vi "test_CCDSetAndGetFitParams.vi"(7 "Test should pass":bool=TRUE, 8 "error in":errorcluster, 9 "tear down connection":bool=TRUE, 10 "set-up a connection":bool=TRUE, 11 "device selection":enum16{"monochromator", "CCD", "SCD"}(ring)=enum."CCD") -> (0 "error out":errorcluster)   [LabVIEW 2023]
uses:
  Classes/CCD/CCD.lvclass
  C:/Projects/Horiba/horiba-labview-sdk/Source/Classes/GenericDevice/GenericDevice.lvclass
  <vilib>/addons/_JKI Toolkits/Caraya/classes/Assert/Assert Equal Value and Type_Variant.vi
  <vilib>/addons/_JKI Toolkits/Caraya/classes/Assert/Assert Not Error.vi
  <vilib>/addons/_JKI Toolkits/Caraya/classes/Assert/Assert Equal Value_Variant.vi
  <vilib>/addons/_JKI Toolkits/Caraya/classes/Test/Test.lvclass
  <vilib>/addons/_JKI Toolkits/Caraya/classes/Assert/Assert.lvclass
panel:
  out "fit parameters":string
  # "Connector Pane"
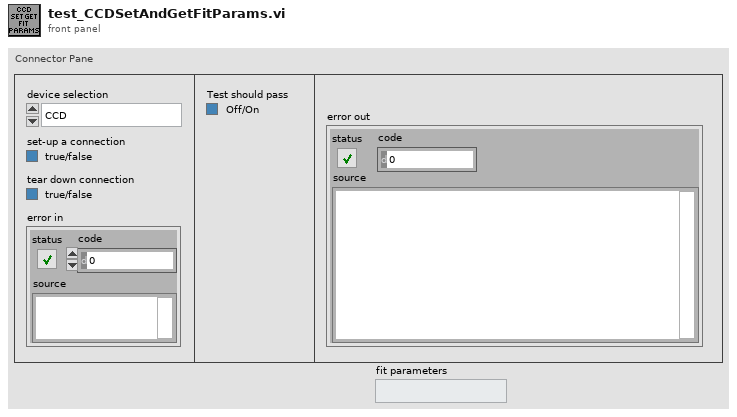
[diagram p1: front panel]
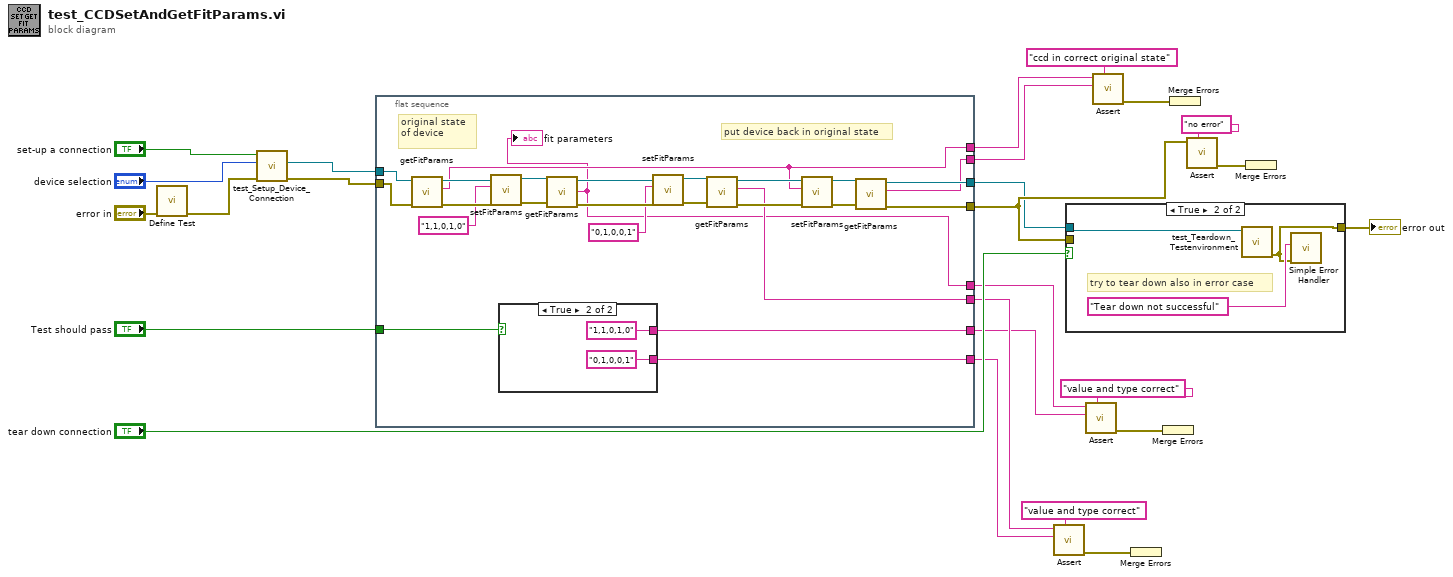
[diagram p0: block diagram]
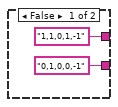
[diagram p2: hidden frame]
diagram:
  n1 = call <vilib>:"Define Test.vi"("error in (no error)"="error in") -> ("error out"=w3:errorcluster)  [unwired: 9 in, 1 out]
  n2 = call "test_Setup_Device_Connection.vi"("error in (no error)"=w3, "device selection"="device selection", "set-up a connection"="set-up a connection") -> ("error out"=w5:errorcluster, "CCD.lvclass"=w4:refnum<class "CCD.lvclass">)  [unwired: 5 in, 2 out]
  n3 = flat-sequence {
    tunnel: w5 -> [w46]
    tunnel: w4 -> [w47]
    tunnel: [w32] -> w16
    tunnel: "Test should pass" -> [w50]
    tunnel: [w39] -> w15
    tunnel: [w27] -> w14
    tunnel: [w49] -> w13
    tunnel: [w26] -> w12
    tunnel: [w48] -> w11
    tunnel: [w30] -> w8
    tunnel: [w31] -> w7
    frame #0 {
      # "put device back in original state"
      # "original state of device"
      n4 = call "getFitParams.vi"("error in (no error)"=w46, "CCD in"=w47) -> ("error out"=w38:errorcluster, "fit parameters"=w30:string, "CCD out"=w45:refnum<class "CCD.lvclass">)  [unwired: 7 in]
      n5 = call "setFitParams.vi"("error in (no error)"=w38, "fit parameters"="1,1,0,1,0", "CCD in"=w45) -> ("error out"=w37:errorcluster, "CCD out"=w44:refnum<class "CCD.lvclass">)  [unwired: 5 in, 2 out]
      n6 = case shown="True" w50 {
        tunnel: ["0,1,0,0,-1" "0,1,0,0,1"] -> w49
        tunnel: ["1,1,0,1,-1" "1,1,0,1,0"] -> w48
        frame False {
        }
        frame True {
        }
      }
      n7 = call "getFitParams.vi"("error in (no error)"=w37, "CCD in"=w44) -> ("error out"=w36:errorcluster, "fit parameters"=w26:string, "CCD out"=w43:refnum<class "CCD.lvclass">)  [unwired: 7 in]
      "fit parameters" <- w26
      n8 = call "setFitParams.vi"("error in (no error)"=w36, "fit parameters"="0,1,0,0,1", "CCD in"=w43) -> ("error out"=w35:errorcluster, "CCD out"=w42:refnum<class "CCD.lvclass">)  [unwired: 5 in, 2 out]
      n9 = call "getFitParams.vi"("error in (no error)"=w35, "CCD in"=w42) -> ("error out"=w34:errorcluster, "fit parameters"=w27:string, "CCD out"=w41:refnum<class "CCD.lvclass">)  [unwired: 7 in]
      n10 = call "setFitParams.vi"("error in (no error)"=w34, "fit parameters"=w30, "CCD in"=w41) -> ("error out"=w33:errorcluster, "CCD out"=w40:refnum<class "CCD.lvclass">)  [unwired: 5 in, 2 out]
      n11 = call "getFitParams.vi"("error in (no error)"=w33, "CCD in"=w40) -> ("error out"=w32:errorcluster, "fit parameters"=w31:string, "CCD out"=w39:refnum<class "CCD.lvclass">)  [unwired: 7 in]
    }
  }
  n12 = call-poly <vilib>:"Assert.vi"("Label"="value and type correct" ("Label (VI Title)"), "Y"=w13, "X"=w14) -> ("error out"=w24:errorcluster)  [unwired: 7 in, 1 out]
  n13 = case shown="True" "tear down connection" {
    tunnel: w15 -> [_ w57]
    tunnel: [w55 w56] -> w6
    tunnel: w16 -> [w55 _]
    frame False {
    }
    frame True {
      # "try to tear down also in error case"
      n14 = call "test_Teardown_Testenvironment.vi"("GenericDevice.lvclass"=w57) -> ("error out"=w56:errorcluster)  [unwired: 9 in, 1 out]
      n15 = call <vilib>:"Simple Error Handler.vi"("error source (\" \")"="Tear down not successful" ("error source (\" \")"), "error in (no error)"=w56) -> ()  [unwired: 3 in, 5 out]
    }
  }
  "error out" <- w6
  n16 = call-poly <vilib>:"Assert.vi"("Label"="value and type correct" ("Label (VI Title)"), "Y"=w11, "X"=w12) -> ("error out"=w23:errorcluster)  [unwired: 7 in, 1 out]
  n17 = call-poly <vilib>:"Assert.vi"("Label"="ccd in correct original state" ("Label (VI Title)"), "Y"=w7, "X"=w8) -> ("error out"=w10:errorcluster)  [unwired: 7 in, 1 out]
  n18 = Merge Errors(w24) -> ()  [unwired: 1 out]
  n19 = Merge Errors(w23) -> ()  [unwired: 1 out]
  n20 = Merge Errors(w10) -> ()  [unwired: 1 out]
  n21 = call-poly <vilib>:"Assert.vi"("Label"="no error" ("Label (VI Title)"), "Not Error?"=w16) -> ("error out"=w18:errorcluster)  [unwired: 8 in, 1 out]
  n22 = Merge Errors(w18) -> ()  [unwired: 1 out]
